vi "HVPPS Current Check.vi"(8 "error in":errorcluster, 10 "WaitMoniter Input":T4={"Wait Time(S)"=10.0, "Chamber Temp(Deg C)"=10.0, "Chamber Temp Tolerance(%)"=10.0, "RMS Current(A)"=10.0, "RMS Current Tolerance(%)"=10.0, "Temperature Control"=FALSE, "RMS Control"=FALSE, "RMS Current Min(A)"=10.0, "RMS Current Max(A)"=10.0, "Chamber Temp Min(Deg C)"=10.0, "Chamber Temp Max(Deg C)"=10.0, "HVPPS Current Max(A)"=10.0, "HVPPS Control"=FALSE, "HVPPS Current(A)"=10.0} {"HVPPS Current(A)" format="%#_13g"; "HVPPS Current Max(A)" format="%#_13g"; "Chamber Temp Max(Deg C)" format="%#_13g"; "Chamber Temp Min(Deg C)" format="%#_13g"; "RMS Current Max(A)" format="%#_13g"; "RMS Current Min(A)" format="%#_13g"; "RMS Current Tolerance(%)" format="%#_13g"; "RMS Current(A)" format="%#_13g"; "Chamber Temp Tolerance(%)" format="%#_13g"; "Chamber Temp(Deg C)" format="%#_13g"; "Wait Time(S)" format="%#_13g"}, 11 "Data Cluster":T1={"Chamber Address"={"Starting Address"=0, "Data Length"=0}, "Modbus RTU"={"unit ID"=1, "serial type"=enum."RTU", "baud rate"=9600, "parity (even)"=2, "flow control (none)"=0, "VISA resource name"=""}, "Temparature PASS?"=FALSE, "RMS Current PASS?"=FALSE, "Ping PASS?"=FALSE, "WaitMonitor_Class"=refnum, "Status Update"="", "Test Mode"=0, "Sequence Context"=refnum, "Running?"=FALSE, "RMS_FAIL_Count"=0, "Current Temperature"=0.0, "Target Temperature"=0.0, "RMS_Current"=[], "PowerStatus"={"Chamber IP Ping"=FALSE, "RAW_Power_Status"=FALSE, "PDU1_Status_Instrument_Rack"=FALSE, "PDU2_Status_PowerSupply_Rack_1"=FALSE, "PDU3_Status_PowerSupply_Rack_2"=FALSE}, "Monitor_Interval(S)"=0.0, "Current_Monitor_Interval(S)"=0.0, "RMS_Refresh?"=FALSE, "RTD Temperature(Deg C)"=0.0, "AbortTime(S)"=0.0, "HVPPS_Current"=[], "HVPPS Current PASS?"=FALSE} {"Modbus RTU"."parity (even)" items=["None", "Odd", "Even", "Mark", "Space"]; "Modbus RTU"."flow control (none)" items=["None", "XON/XOFF", "RTS/CTS", "XON/XOFF & RTS/CTS", "DTR/DSR", "XON/XOFF & DTR/DSR"]}) -> (0 "error out":errorcluster, 3 "Data Cluster out":T1={"Chamber Address"={"Starting Address"=0, "Data Length"=0}, "Modbus RTU"={"unit ID"=1, "serial type"=enum."RTU", "baud rate"=9600, "parity (even)"=2, "flow control (none)"=0, "VISA resource name"=""}, "Temparature PASS?"=FALSE, "RMS Current PASS?"=FALSE, "Ping PASS?"=FALSE, "WaitMonitor_Class"=refnum, "Status Update"="", "Test Mode"=0, "Sequence Context"=refnum, "Running?"=FALSE, "RMS_FAIL_Count"=0, "Current Temperature"=0.0, "Target Temperature"=0.0, "RMS_Current"=[], "PowerStatus"={"Chamber IP Ping"=FALSE, "RAW_Power_Status"=FALSE, "PDU1_Status_Instrument_Rack"=FALSE, "PDU2_Status_PowerSupply_Rack_1"=FALSE, "PDU3_Status_PowerSupply_Rack_2"=FALSE}, "Monitor_Interval(S)"=0.0, "Current_Monitor_Interval(S)"=0.0, "RMS_Refresh?"=FALSE, "RTD Temperature(Deg C)"=0.0, "AbortTime(S)"=0.0, "HVPPS_Current"=[], "HVPPS Current PASS?"=FALSE} {"Modbus RTU"."parity (even)" items=["None", "Odd", "Even", "Mark", "Space"]; "Modbus RTU"."flow control (none)" items=["None", "XON/XOFF", "RTS/CTS", "XON/XOFF & RTS/CTS", "DTR/DSR", "XON/XOFF & DTR/DSR"]})   [LabVIEW 2023, in "HardwareAbstractionLayer_LVOOP.lvlib" / "Wait Monitor.lvclass"]
uses:
  Wait Monitor.lvclass
  Teststand Steptypes/WaitMoniter/Control/Moniter Step Control.ctl
  Control/Data Cluster.ctl
  <vilib>/addons/TestStand/_TSLegacy.llb/LabVIEW Test - Sequence Context.ctl
  Teststand Steptypes/PowerMonitor/Control/PowerData.ctl
  PowerSupply/Control/PPS FGV Option.ctl
  <vilib>/addons/TestStand/_TSUtility.llb/TestStand - Get Property Value (Number).vi
  PowerSupply/PowerSupply.lvclass
  Wait Monitor.lvclass/Wait Monitor.ctl
  Teststand/Teststand.lvclass
  <userlib>/_OpenG.lib/error/error.llb/openg_error.lvlib
  Teststand Steptypes/LTT_TeststandSteptypes.lvlib
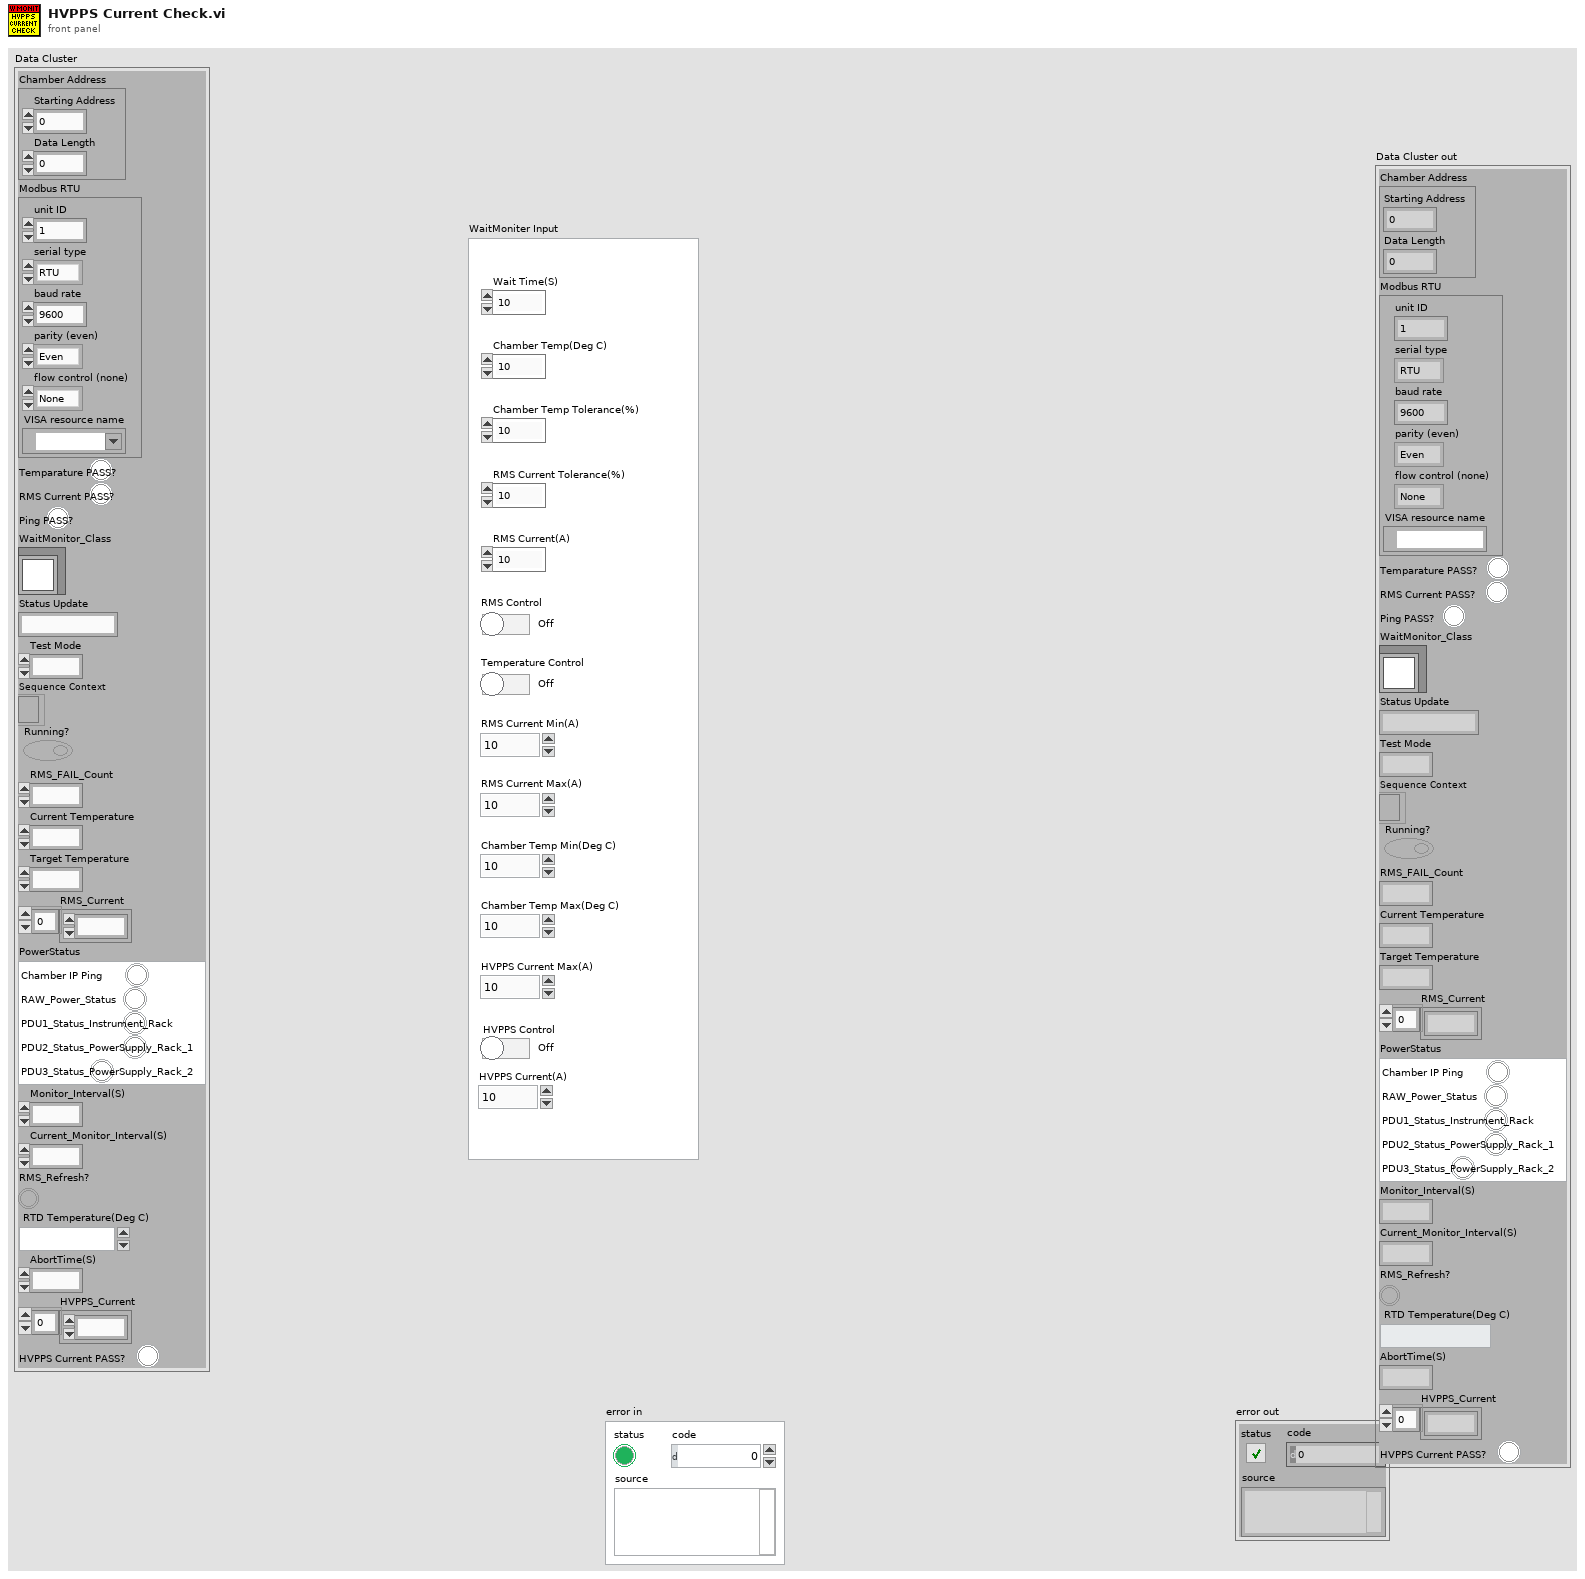
[diagram p1: front panel]
types:
  T1 = typedef "HardwareAbstractionLayer_LVOOP.lvlib/Wait Monitor.lvclass/Data Cluster.ctl" = cluster{"Chamber Address":cluster{"Starting Address":u16, "Data Length":u16}, "Modbus RTU":cluster{"unit ID":u8, "serial type":enum16{"RTU", "ASCII"}, "baud rate":u32, "parity (even)":u16, "flow control (none)":u16, "VISA resource name":refnum<visa-resource-name>}, "Temparature PASS?":bool, "RMS Current PASS?":bool, "Ping PASS?":bool, "WaitMonitor_Class":refnum<class "Wait Monitor.lvclass">, "Status Update":string, "Test Mode":u16, "Sequence Context":T2, "Running?":bool, "RMS_FAIL_Count":u16, "Current Temperature":dbl, "Target Temperature":dbl, "RMS_Current":dbl[], "PowerStatus":T3, "Monitor_Interval(S)":dbl, "Current_Monitor_Interval(S)":dbl, "RMS_Refresh?":bool, "RTD Temperature(Deg C)":dbl, "AbortTime(S)":dbl, "HVPPS_Current":dbl[], "HVPPS Current PASS?":bool}
  T2 = typedef "LabVIEW Test - Sequence Context.ctl" = refnum<k7>
  T3 = typedef "LTT_TeststandSteptypes.lvlib/PowerData.ctl" = cluster{"Chamber IP Ping":bool, "RAW_Power_Status":bool, "PDU1_Status_Instrument_Rack":bool, "PDU2_Status_PowerSupply_Rack_1":bool, "PDU3_Status_PowerSupply_Rack_2":bool}
  T4 = typedef "HardwareAbstractionLayer_LVOOP.lvlib/Wait Monitor.lvclass/Moniter Step Control.ctl" = cluster{"Wait Time(S)":dbl, "Chamber Temp(Deg C)":dbl, "Chamber Temp Tolerance(%)":dbl, "RMS Current(A)":dbl, "RMS Current Tolerance(%)":dbl, "Temperature Control":bool, "RMS Control":bool, "RMS Current Min(A)":dbl, "RMS Current Max(A)":dbl, "Chamber Temp Min(Deg C)":dbl, "Chamber Temp Max(Deg C)":dbl, "HVPPS Current Max(A)":dbl, "HVPPS Control":bool, "HVPPS Current(A)":dbl}
  T5 = typedef "HardwareAbstractionLayer_LVOOP.lvlib/PowerSupply.lvclass/PPS FGV Option.ctl" = enum16{"Init Ref", "Get Ref", "Set Ref"}
  T6 = typedef "HardwareAbstractionLayer_LVOOP.lvlib/Teststand.lvclass/Teststand Status Control.ctl" = cluster{"Terminating or Aborting":bool, "Stop":bool, "Socket Count":i16, "Selected Sockets":i16[]}
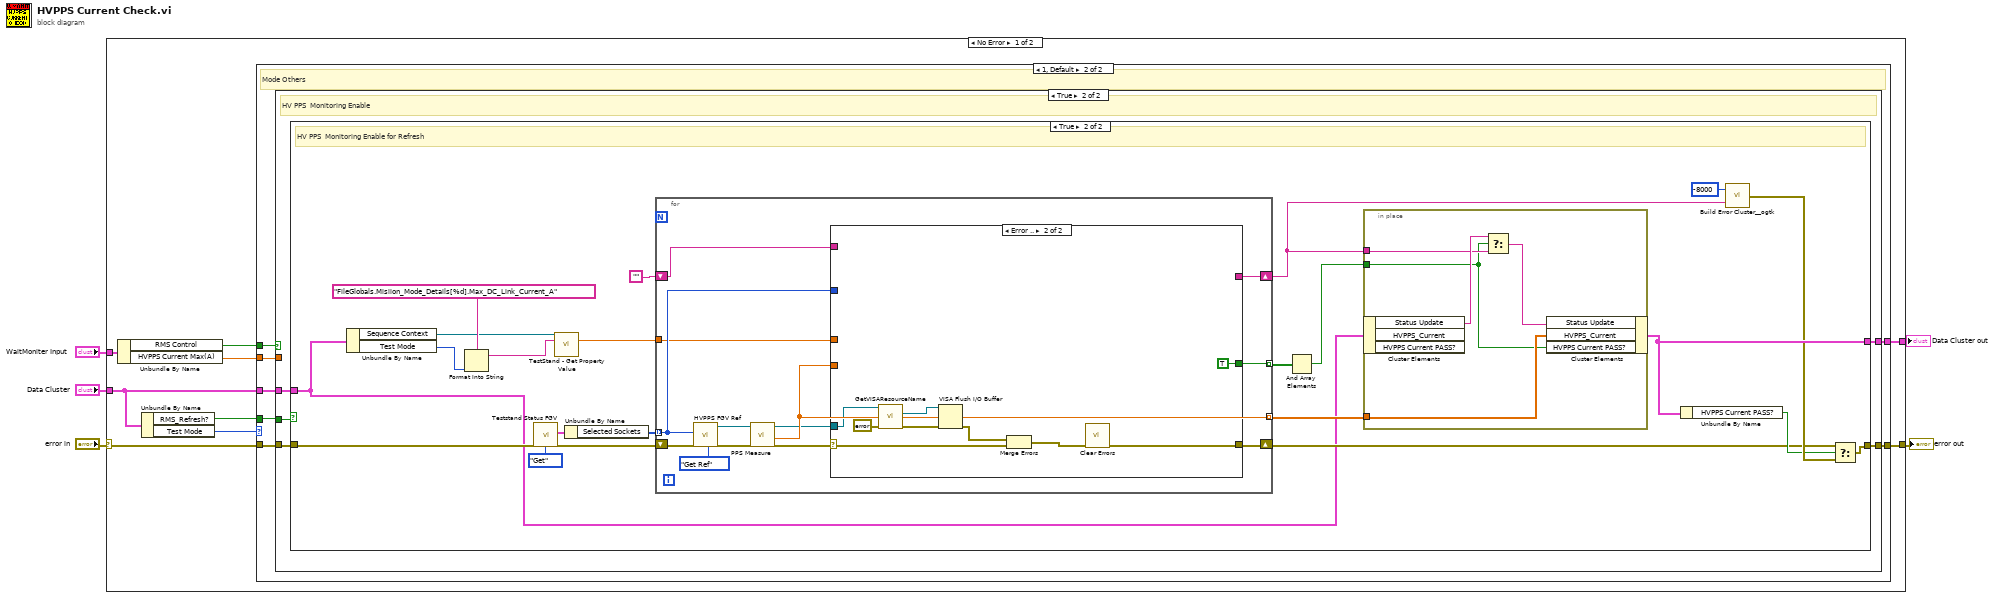
[diagram p0: block diagram]
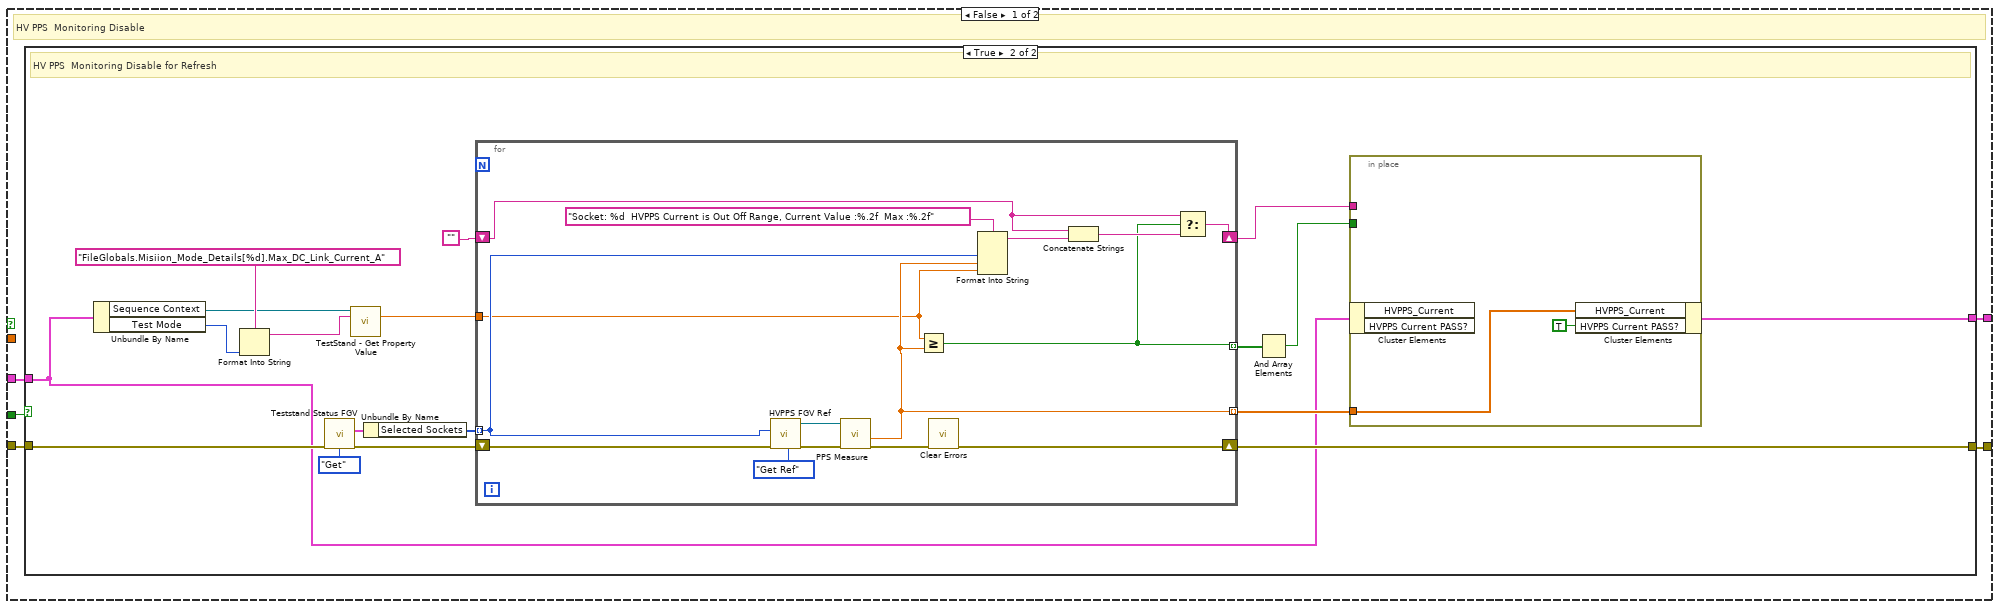
[diagram p3: hidden frame]
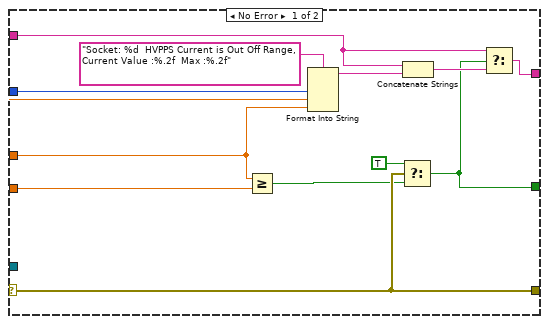
[diagram p6: hidden frame]
diagram:
  n1 = case shown="No Error" "error in" {
    selector: "error in" -> [w14 w135]
    tunnel: [w13 w135] -> w4
    tunnel: "WaitMoniter Input" -> [w12 _]
    tunnel: "Data Cluster" -> [w8 w134]
    tunnel: [w11 w134] -> w1
    frame No Error {
      n2 = Unbundle By Name(w12) -> ("RMS Control"=w9:bool, "HVPPS Current Max(A)"=w10:dbl)
      n3 = Unbundle By Name(w8) -> ("RMS_Refresh?"=w7:bool, "Test Mode"=w6:u16)
      n4 = case shown="1, Default" w6 {
        tunnel: w14 -> [w15 w23]
        tunnel: [w15 w22] -> w13
        tunnel: [w16 w21] -> w11
        tunnel: w10 -> [_ w20]
        tunnel: w9 -> [_ w19]
        tunnel: w8 -> [w16 w18]
        tunnel: w7 -> [_ w17]
        frame 0 {
          # "Mode 0"
        }
        frame 1, Default {
          # "Mode Others"
          n5 = case shown="True" w19 {
            tunnel: w23 -> [w26 w70]
            tunnel: [w24 w68] -> w22
            tunnel: w18 -> [w28 w67]
            tunnel: [w25 w69] -> w21
            tunnel: w20 -> [_ _]
            tunnel: w17 -> [w27 w66]
            frame False {
              # "HV PPS  Monitoring Disable"
              n6 = case shown="True" w27 {
                tunnel: w26 -> [w29 w48]
                tunnel: [w30 w47] -> w25
                tunnel: [w29 w37] -> w24
                tunnel: w28 -> [w30 w34]
                frame False {
                  # "HV PPS  Monitoring Disable for not Refresh"
                }
                frame True {
                  # "HV PPS  Monitoring Disable for Refresh"
                  n7 = Unbundle By Name(w34) -> ("Sequence Context"=w33:T2, "Test Mode"=w32:u16)
                  n8 = Format Into String(format string="FileGlobals.Misiion_Mode_Details[%d].Max_DC_Link_Current_A" ("Lookup String"), w32) -> (resulting string=w36:string)  [unwired: 2 in, 1 out]
                  n9 = call "Teststand Status FGV.vi"("error in"=w48, "Option"=enum16{"Set", "Get"}."Get") -> ("error out"=w43:errorcluster, "Teststand Status Out"=w45:T6)  [unwired: 8 in]
                  n10 = call-poly <vilib>:"TestStand - Get Property Value.vi"("Sequence Context In"=w33, "Lookup String"=w36) -> ("Value"=w31:dbl)  [unwired: 11 in, 2 out]
                  n11 = Unbundle By Name(w45) -> ("Selected Sockets"=w44:i16[])
                  n12 = for {
                    tunnel: w44 -> [w58] mode=indexing
                    shift-right: [w51] -> w37
                    shift-left: w43 -> [w65]
                    tunnel: [w54] -> w42 mode=indexing
                    shift-right: [w62] -> w39
                    shift-left: "" -> [w60]
                    tunnel: [w53] -> w38 mode=indexing
                    tunnel: w31 -> [w52]
                    n13 = call "HVPPS FGV Ref.vi"("Option"=PPS_FGV_Option."Get Ref", "error in"=w65, "Socket No"=w58) -> ("error out"=w56:errorcluster, "PowerSupplyOut.lvclass"=w57:refnum<class "PowerSupply.lvclass">)  [unwired: 7 in]
                    n14 = call-dynamic "PPS Measure.vi"("error in (no error)"=w56, "PowerSupply in"=w57) -> ("error out"=w55:errorcluster, "Actual Current Limit (A)"=w53:dbl)  [unwired: 6 in, 2 out]
                    n15 = Greater Or Equal?(x=w52, y=w53) -> (x >= y?=w54:bool)
                    n16 = call <vilib>:"Clear Errors.vi"("error in (no error)"=w55) -> ("error out"=w51:errorcluster)  [unwired: 5 in, 1 out]
                    n17 = Format Into String(format string="Socket: %d  HVPPS Current is Out Off Range, Current Value :%.2f  Max :%.2f", w58, w53, w52) -> (resulting string=w63:string)  [unwired: 2 in, 1 out]
                    n18 = Concatenate Strings(w60, w63) -> (w61:string)
                    n19 = Select(t=w60, s=w54, f=w61) -> (s? t:f=w62:string)
                  }
                  n20 = And Array Elements(Boolean array=w42) -> (logical AND=w41:bool)
                  n21 = in-place {
                    in-place-border: w41 -> [_]
                    in-place-border: w39 -> [_]
                    in-place-border: w38 -> [w50]
                    n22 = in-place-cluster #1(w34) -> ()  [unwired: 2 out]
                    n23 = in-place-cluster #1("HVPPS_Current"=w50, "HVPPS Current PASS?"=TRUE) -> (w47:T1)
                  }
                }
              }
            }
            frame True {
              # "HV PPS  Monitoring Enable"
              n24 = case shown="True" w66 {
                tunnel: w70 -> [w71 w94]
                tunnel: [w72 w93] -> w69
                tunnel: [w71 w92] -> w68
                tunnel: w67 -> [w72 w76]
                frame False {
                  # "HV PPS  Monitoring Enable for not refresh"
                }
                frame True {
                  # "HV PPS  Monitoring Enable for Refresh"
                  n25 = Unbundle By Name(w76) -> ("Sequence Context"=w75:T2, "Test Mode"=w74:u16)
                  n26 = Format Into String(format string="FileGlobals.Misiion_Mode_Details[%d].Max_DC_Link_Current_A" ("Lookup String"), w74) -> (resulting string=w78:string)  [unwired: 2 in, 1 out]
                  n27 = call "Teststand Status FGV.vi"("error in"=w94, "Option"=enum16{"Set", "Get"}."Get") -> ("error out"=w88:errorcluster, "Teststand Status Out"=w90:T6)  [unwired: 8 in]
                  n28 = call-poly <vilib>:"TestStand - Get Property Value.vi"("Sequence Context In"=w75, "Lookup String"=w78) -> ("Value"=w73:dbl)  [unwired: 11 in, 2 out]
                  n29 = Unbundle By Name(w90) -> ("Selected Sockets"=w89:i16[])
                  n30 = for {
                    tunnel: w89 -> [w108] mode=indexing
                    shift-right: [w103] -> w79
                    shift-left: w88 -> [w112]
                    tunnel: [w101] -> w87 mode=indexing
                    shift-right: [w111] -> w84
                    shift-left: "" -> [w110]
                    tunnel: [w105] -> w82 mode=indexing
                    tunnel: w73 -> [w104]
                    n31 = call "HVPPS FGV Ref.vi"("Option"=PPS_FGV_Option."Get Ref", "error in"=w112, "Socket No"=w108) -> ("error out"=w106:errorcluster, "PowerSupplyOut.lvclass"=w107:refnum<class "PowerSupply.lvclass">)  [unwired: 7 in]
                    n32 = call-dynamic "PPS Measure.vi"("error in (no error)"=w106, "PowerSupply in"=w107) -> ("error out"=w102:errorcluster, "Actual Current Limit (A)"=w105:dbl, "PowerSupply out"=w100:refnum<class "PowerSupply.lvclass">)  [unwired: 6 in, 1 out]
                    n33 = case shown="Error .." w102 {
                      selector: w102 -> [w116 w133]
                      tunnel: [w122 _] -> w111
                      tunnel: w110 -> [w120 _]
                      tunnel: w108 -> [w119 _]
                      tunnel: w105 -> [w118 _]
                      tunnel: w104 -> [w117 _]
                      tunnel: [w116 w132] -> w103
                      tunnel: [w114 TRUE ("t")] -> w101
                      tunnel: w100 -> [_ w130]
                      frame No Error {
                        n34 = Greater Or Equal?(x=w117, y=w118) -> (x >= y?=w115:bool)
                        n35 = Format Into String(format string="Socket: %d  HVPPS Current is Out Off Range, Current Value :%.2f  Max :%.2f", w119, w118, w117) -> (resulting string=w123:string)  [unwired: 2 in, 1 out]
                        n36 = Select(t=TRUE, s=w116, f=w115) -> (s? t:f=w114:bool)
                        n37 = Concatenate Strings(w120, w123) -> (w121:string)
                        n38 = Select(t=w120, s=w114, f=w121) -> (s? t:f=w122:string)
                      }
                      frame Error {
                        n39 = call "GetVISAResourceName.vi"("error in (no error)"=errorcluster {"status"=FALSE, "code"=0, "source"=""}, "object in"=w130) -> ("error out"=w126:errorcluster, "VISA resource name"=w127:refnum<visa-resource-name>)  [unwired: 7 in, 1 out]
                        n40 = VISA Flush I/O Buffer(VISA resource name=w127, error in (no error)=w126) -> (error out=w125:errorcluster)  [unwired: 1 in, 1 out]
                        n41 = Merge Errors(w125, w133) -> (w129:errorcluster)
                        n42 = call <vilib>:"Clear Errors.vi"("error in (no error)"=w129) -> ("error out"=w132:errorcluster)  [unwired: 5 in, 1 out]
                      }
                    }
                  }
                  n43 = And Array Elements(Boolean array=w87) -> (logical AND=w86:bool)
                  n44 = in-place {
                    in-place-border: w86 -> [w95]
                    in-place-border: w84 -> [w98]
                    in-place-border: w82 -> [w96]
                    n45 = in-place-cluster #2(w76) -> ("Status Update"=w99:string)  [unwired: 2 out]
                    n46 = Select(t=w99, s=w95, f=w98) -> (s? t:f=w97:string)
                    n47 = in-place-cluster #2("Status Update"=w97, "HVPPS_Current"=w96, "HVPPS Current PASS?"=w95) -> (w93:T1)
                  }
                  n48 = Unbundle By Name(w93) -> ("HVPPS Current PASS?"=w80:bool)
                  n49 = call <userlib>:"Build Error Cluster__ogtk.vi"("String to Prepend to source (\"\")"=w84, "code"=-8000) -> ("error out"=w81:errorcluster)
                  n50 = Select(t=w79, s=w80, f=w81) -> (s? t:f=w92:errorcluster)
                }
              }
            }
          }
        }
      }
    }
    frame Error {
    }
  }
  "error out" <- w4
  "Data Cluster out" <- w1
